vi "FPGA_main_simplified.vi"() -> ()   [LabVIEW 2020]
uses:
  <vilib>/Platform/TimedLoop/XDataNode/timing_clust.ctl
  <vilib>/Platform/TimedLoop/XDataNode/nitl_modes.ctl
  <vilib>/Platform/TimedLoop/XDataNode/wakeup.ctl
  <vilib>/LabVIEW Targets/FPGA/cRIO/shared/nicrio_ModuleControls/nicrio_cRIO-9775_ContinuousDataRates4ChansRing.ctl
  <vilib>/rvi/Emulation/niFpgaGetClockAttributes.vi
  <vilib>/rvi/Emulation/niFpgaSctlEmulationGetInTimedLoop.vi
  <vilib>/rvi/Emulation/niFpgaEmulationReportErrorSimple.vi
  <vilib>/rvi/Emulation/niFpgaProcessEmulError.vi
  <vilib>/rvi/Emulation/niFpgaCriticalErrorInLSC.vi
  <vilib>/rvi/eio/common/nirviEmuTemplateMethod_errors.vi
  <vilib>/rvi/eio/common/nirviEmuTemplatePropertySet_errors.vi
  <vilib>/rvi/interface/RandomDataEmulation/niFpgaRandomDataHandleErrors.vi
  <vilib>/platform/TimedLoop/XDataNode/XDataNode.xnode
  <vilib>/eio/EIONode/EIONode.xnode
  <vilib>/eio/EIOMethodNode/EIOMethodNode.xnode
  <vilib>/eio/EIOPropertyNode/EIOPropertyNode.xnode
  <vilib>/rvi/DataTransferAndStorage/Container/XNode/niFpgaContainer.xnode
  <vilib>/rvi/interface/RandomDataEmulation/nirviRandomDataFpgaReadWriteTemplate.vi
  <vilib>/Platform/TimedLoop/XDataNode/XDNodeRunTimeDep.lvlib
  <vilib>/rvi/eio/common/nirviEmuTemplatePropertyGet_errors.vi
  <vilib>/rvi/eio/common/nirviEmuTemplatePropertyGet_noerrors.vi
  <vilib>/rvi/eio/common/nirviEmuTemplatePropertySet_noerrors.vi
panel:
  out "FPGA routine\nrunning":bool
  in  "Pulse\nWidth":u32 caption="Pulse width(uSec)"
  in  "Pulse\nPeriod":u32 caption="Period(uSec)"
  in  "Stop Routine":bool
  in  "DIO3":bool
  in  "DIO2":bool
  in  "DIO1":bool
  in  "DIO0":bool
  out "Rebinned Counts":i32
  in  "Binning Time (ticks)":i32=1200000
  out "Counts":u8
  out "FPGA Error":errorcluster
  out "Finished":bool
  in  "Stop":bool
  out "Module Underflow":bool
  out "DMA FIFO Full":bool
  out "Actual Loop Period (ticks)":u32=40
  out "First Read":bool
  in  "Type Counter":enum16{"Falling Edge", "Rising Edge"}(ring)
  # "Photon counting. Single cycle time loop"
  # "User Control of digital output"
  # "Thresholding"
  # "Pulsing DIO 0 (Pulse width should be shorter than\n period)"
  # "Binning and streaming binned Total Count"
  # "Streaming Analog Input Data"
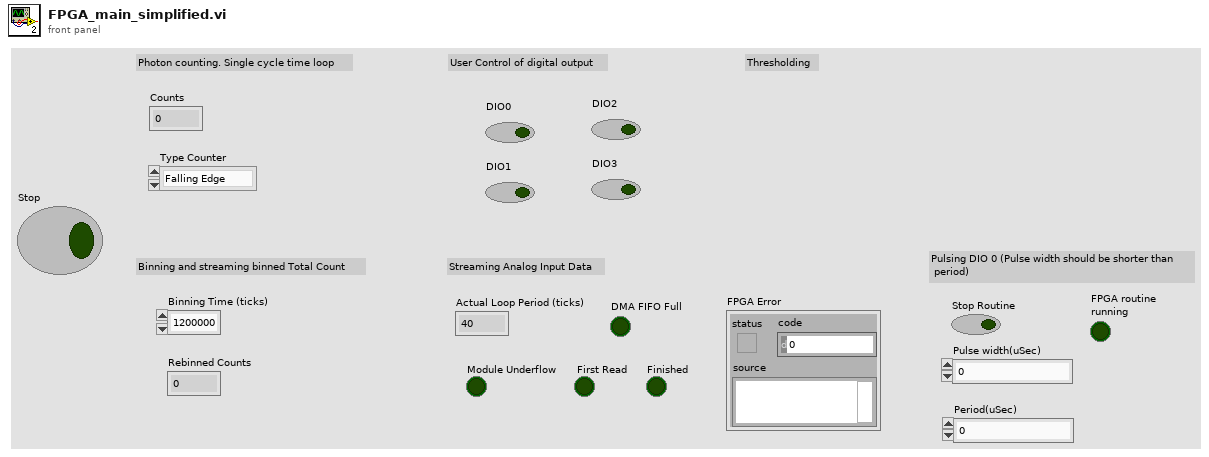
[diagram p1: front panel]
types:
  T1 = typedef "nicrio_cRIO-9775_ContinuousDataRates4ChansRing.ctl" = u16
  T2 = typedef "XDNodeRunTimeDep.lvlib/timing_clust.ctl" = cluster{"Expected End [f-1]":u64, "Actual End [f-1]":u64, "Finished Late? [f-1]":bool, "Expected End [i-1]":u64, "Actual End [i-1]":u64, "Finished Late? [i-1]":bool, "Expected Start [i]":u64, "Actual Start [i]":u64, "Expected Start [f]":u64, "Actual Start [f]":u64, "Source Name":string, "Structure Name":string, "Period":i64, "Deadline":i64, "Offset":i64, "Start":i64, "Priority":i32, "Timeout":i32, "Mode":T3, "Wakeup Reason":T4, "Error":errorcluster, "Source Type":string, "Secondary Source Type":string, "Global End Time":u64, "Global Start Time":u64, "Frame Duration":u64, "Iteration Duration":u64, "Assigned CPU":i32, "I/O Scan Engine Mode":u32}
  T3 = typedef "XDNodeRunTimeDep.lvlib/nitl_modes.ctl" = enum32{"No Change", "Process missed periods, maintain original phase", "Discard missed periods, maintain original phase", "Process missed periods, ignore original phase", "Discard missed periods, ignore original phase"}
  T4 = typedef "XDNodeRunTimeDep.lvlib/wakeup.ctl" = enum32{"Normal", "Aborted", "Asynchronous wakeup", "Timing source error", "Timed loop error", "Timeout"}
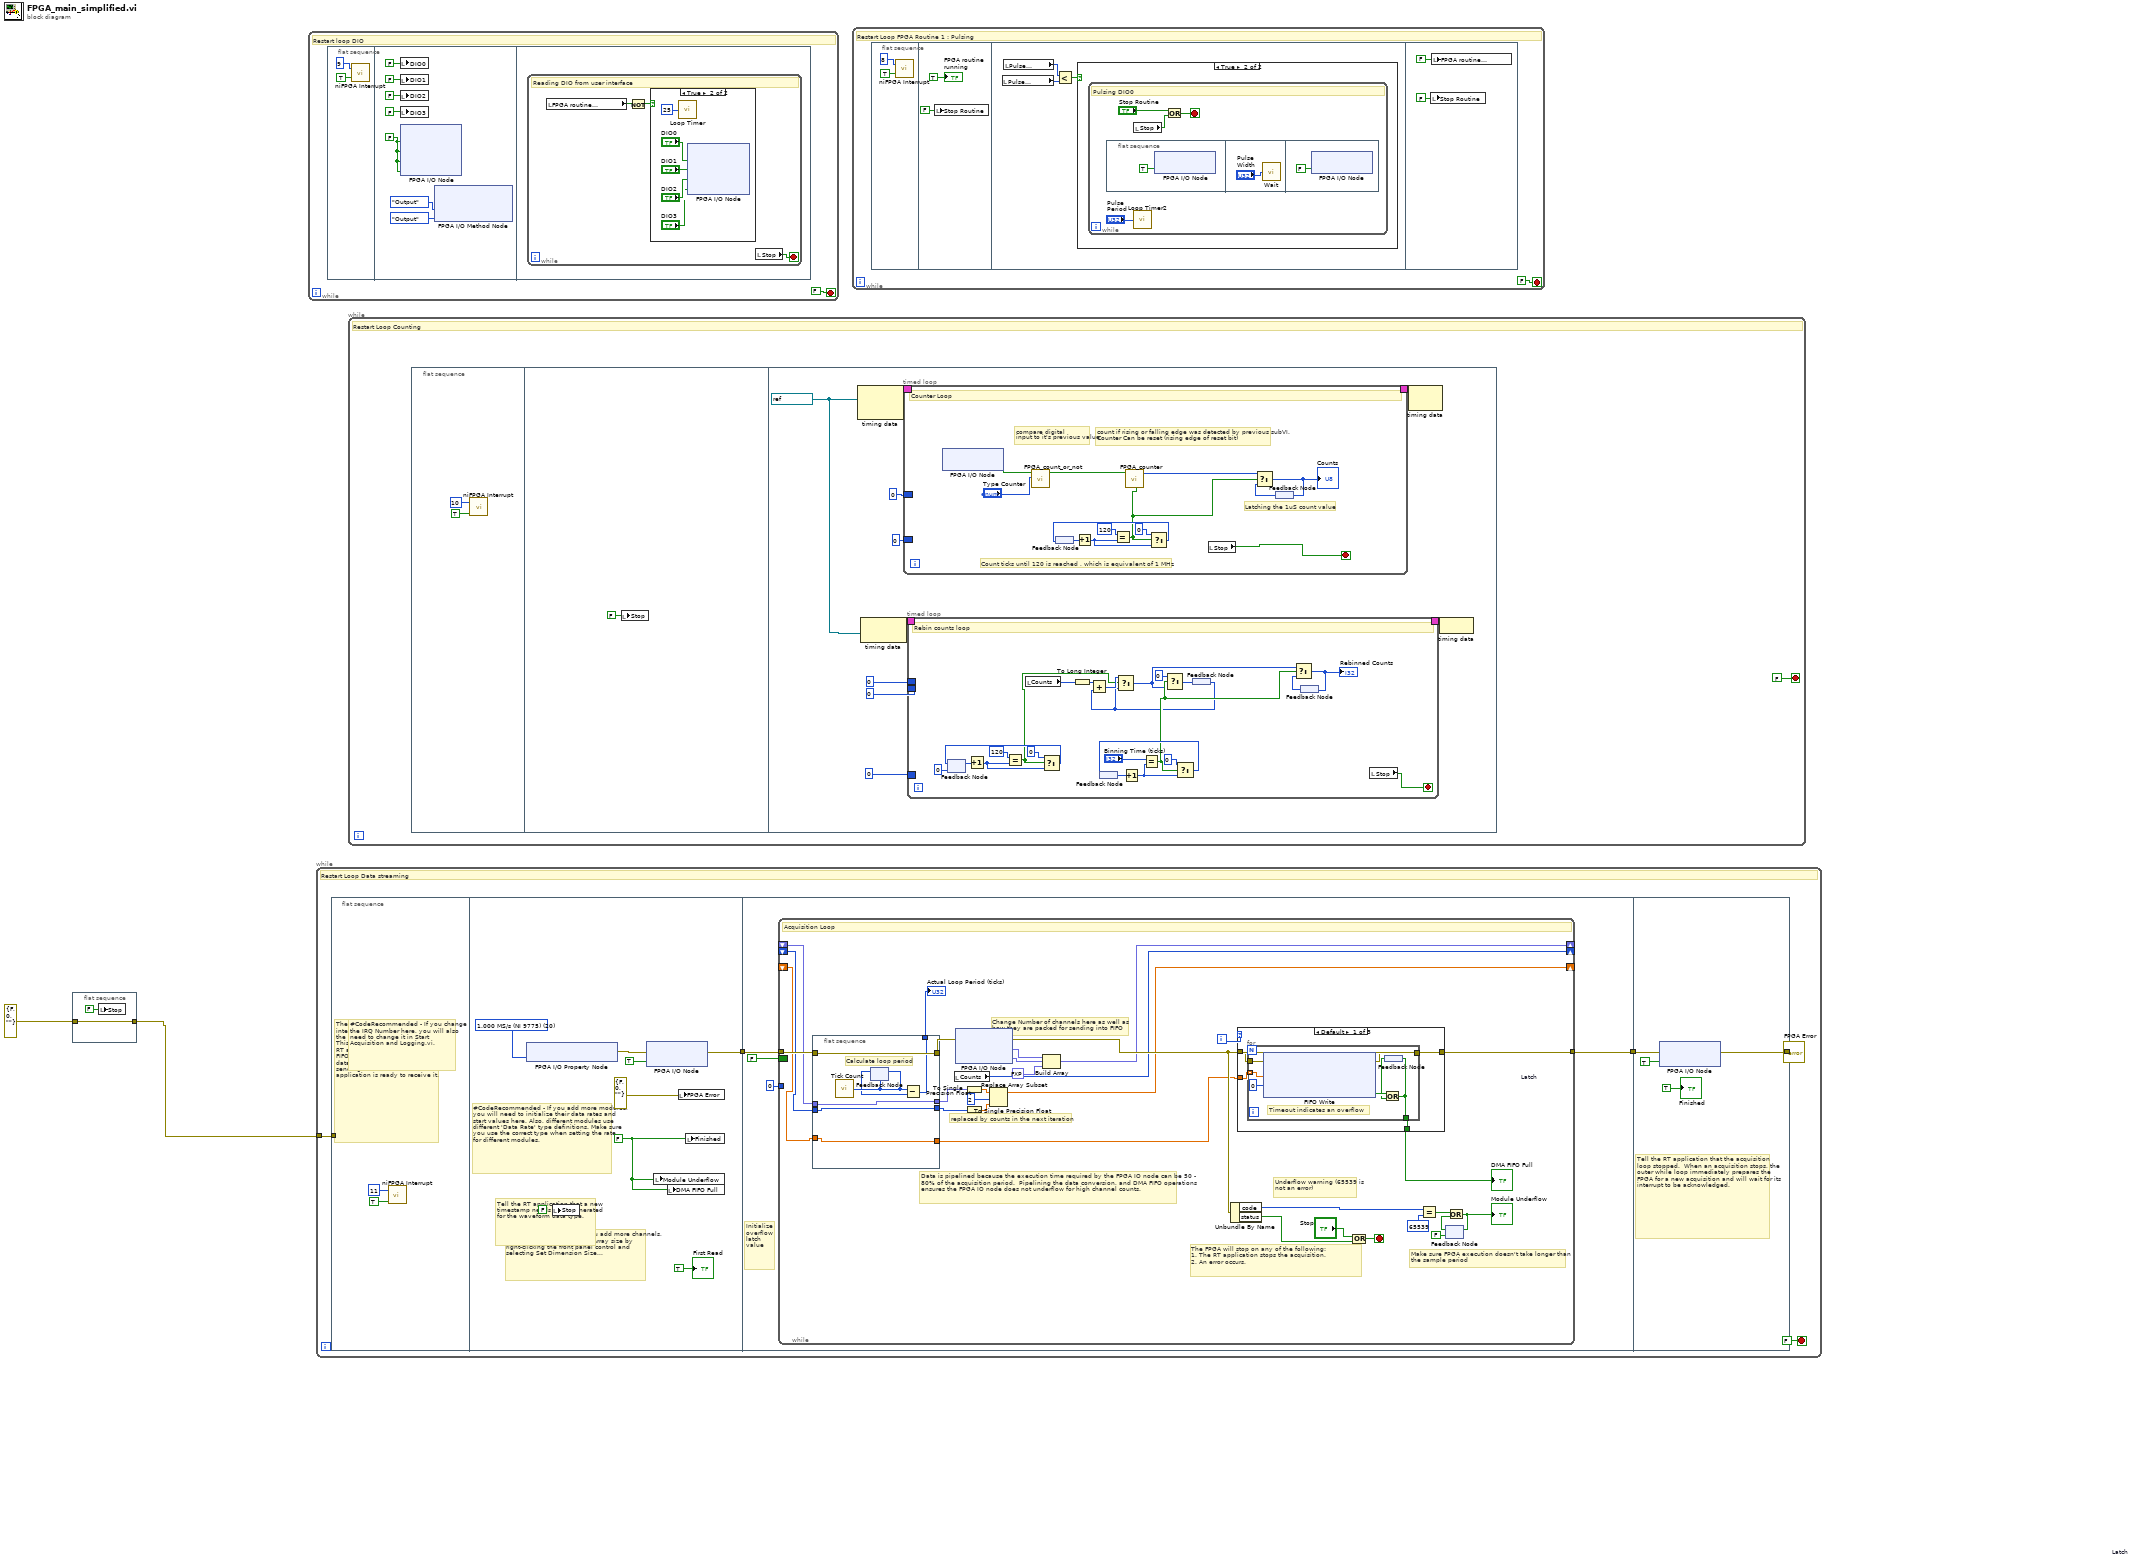
[diagram p0: block diagram]
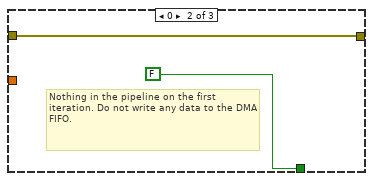
[diagram p4: hidden frame]
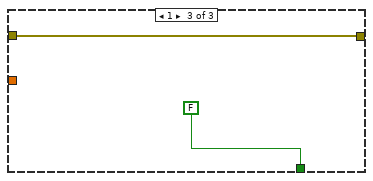
[diagram p5: hidden frame]
diagram:
  n1 = flat-sequence {
    tunnel: errorcluster {"status"=FALSE, "code"=0, "source"=""} ("Error") -> [w3]
    tunnel: [w3] -> w1
    frame #0 {
      n2 = local write "Stop"(FALSE ("stop")) -> ()
    }
  }
  n3 = while {
    stop <- FALSE stop-if-true
    # "Restart loop DIO"
    n4 = flat-sequence {
      frame #0 {
        n5 = call <vilib>:"niFPGA Interrupt.vi"("Wait Until Cleared (F)"=TRUE ("Wait Until Cleared"), "IRQ Number (0)"=u8 9 ("IRQ Number")) -> ()  [unwired: 1 in]
      }
      frame #1 {
        w10 = FALSE ("Mod3/DIO0")
        n6 = local write "DIO0"(FALSE ("DIO0")) -> ()
        n7 = local write "DIO1"(FALSE ("DIO1")) -> ()
        n8 = local write "DIO2"(FALSE ("DIO2")) -> ()
        n9 = local write "DIO3"(FALSE ("DIO3")) -> ()
        n10 = xnode "FPGA I/O Node"("Mod3/DIO0"=w10, "Mod3/DIO1"=w10, "Mod3/DIO2"=w10, "Mod3/DIO3"=w10) -> ()  [unwired: 4 in, 4 out]
        n11 = xnode "FPGA I/O Method Node"("DIO 7:4"=enum8{"No Change", "Input", "Output"}."Output", "DIO 3:0"=enum8{"No Change", "Input", "Output"}."Output") -> ()  [unwired: 1 in, 1 out]
      }
      frame #2 {
        n12 = while {
          stop <- w17 stop-if-true
          # "Reading DIO from user interface"
          n13 = local read "FPGA routine\nrunning"() -> (w16:bool)
          n14 = Not(x=w16) -> (.not. x?=w15:bool)
          n15 = case shown="True" w15 {
            frame False {
            }
            frame True {
              n16 = call "Loop Timer"("Count(mSec)"=u8 25) -> ()  [unwired: 1 out]
              n17 = xnode "FPGA I/O Node"("Mod3/DIO0"="DIO0", "Mod3/DIO1"="DIO1", "Mod3/DIO2"="DIO2", "Mod3/DIO3"="DIO3") -> ()  [unwired: 4 in, 4 out]
            }
          }
          n18 = local read "Stop"() -> (w17:bool)
        }
      }
    }
  }
  n19 = while {
    tunnel: w1 -> [w23]
    stop <- FALSE stop-if-true
    # "Restart Loop Data streaming"
    n20 = flat-sequence {
      tunnel: w23 -> [_]
      tunnel: [w37] -> w26
      tunnel: w26 -> [w39]
      tunnel: [w38] -> w25
      tunnel: w25 -> [w96]
      tunnel: [w95] -> w24
      frame #0 {
        # "#CodeRecommended - If you change the IRQ Number here, you will also need to change it in Start Acquisition and Logging.vi."
        # "The RT application waits on this interrupt to synchronize itself with the start of the FPGA's acquisition.  This synchronization prevents the RT application from polling the DMA FIFO before the FPGA is sending its data. It also prevents the FPGA from sending its data before the RT application is ready to receive it."
        n21 = call <vilib>:"niFPGA Interrupt.vi"("Wait Until Cleared (F)"=TRUE ("Wait Until Cleared"), "IRQ Number (0)"=u8 11 ("IRQ Number")) -> ()  [unwired: 1 in]
      }
      frame #1 {
        w31 = T1 20 items=["1.000 MS/s (NI 9775)"=20, "833.333 KS/s (NI 9775)"=24, "714.286 KS/s (NI 9775)"=28, "625.000 KS/s (NI 9775)"=32, "555.556 KS/s (NI 9775)"=36, "500.000 KS/s (NI 9775)"=40, "454.545 KS/s (NI 9775)"=44, "416.667 KS/s (NI 9775)"=48, "384.615 KS/s (NI 9775)"=52, "357.143 KS/s (NI 9775)"=56, "333.333 KS/s (NI 9775)"=60, "312.500 KS/s (NI 9775)"=64, "294.118 KS/s (NI 9775)"=68, "277.778 KS/s (NI 9775)"=72, "263.158 KS/s (NI 9775)"=76, "250.000 KS/s (NI 9775)"=80, "238.095 KS/s (NI 9775)"=84, "227.273 KS/s (NI 9775)"=88, "217.391 KS/s (NI 9775)"=92, "208.333 KS/s (NI 9775)"=96, "200.000 KS/s (NI 9775)"=100, "192.308 KS/s (NI 9775)"=104, "185.185 KS/s (NI 9775)"=108, "178.571 KS/s (NI 9775)"=112, "172.414 KS/s (NI 9775)"=116, "166.667 KS/s (NI 9775)"=120, "161.290 KS/s (NI 9775)"=124, "156.250 KS/s (NI 9775)"=128, "151.515 KS/s (NI 9775)"=132, "147.059 KS/s (NI 9775)"=136, "142.857 KS/s (NI 9775)"=140, "138.889 KS/s (NI 9775)"=144, "135.135 KS/s (NI 9775)"=148, "131.579 KS/s (NI 9775)"=152, "128.205 KS/s (NI 9775)"=156, "125.000 KS/s (NI 9775)"=160, "121.951 KS/s (NI 9775)"=164, "119.048 KS/s (NI 9775)"=168, "116.279 KS/s (NI 9775)"=172, "113.636 KS/s (NI 9775)"=176, "111.111 KS/s (NI 9775)"=180, "108.696 KS/s (NI 9775)"=184, "106.383 KS/s (NI 9775)"=188, "104.167 KS/s (NI 9775)"=192, "102.041 KS/s (NI 9775)"=196, "100.000 KS/s (NI 9775)"=200, "50.000 KS/s (NI 9775)"=400, "33.333 KS/s (NI 9775)"=600, "25.000 KS/s (NI 9775)"=800, "20.000 KS/s (NI 9775)"=1000, "16.667 KS/s (NI 9775)"=1200, "14.286 KS/s (NI 9775)"=1400, "12.500 KS/s (NI 9775)"=1600, "11.111 KS/s (NI 9775)"=1800, "10.000 KS/s (NI 9775)"=2000, "9.091 KS/s (NI 9775)"=2200, "8.333 KS/s (NI 9775)"=2400, "7.692 KS/s (NI 9775)"=2600, "7.143 KS/s (NI 9775)"=2800, "6.667 KS/s (NI 9775)"=3000, "6.250 KS/s (NI 9775)"=3200, "5.882 KS/s (NI 9775)"=3400, "5.556 KS/s (NI 9775)"=3600, "5.000 KS/s (NI 9775)"=4000, "4.762 KS/s (NI 9775)"=4200, "4.545 KS/s (NI 9775)"=4400, "4.348 KS/s (NI 9775)"=4600, "4.167 KS/s (NI 9775)"=4800, "4.000 KS/s (NI 9775)"=5000, "3.846 KS/s (NI 9775)"=5200, "3.571 KS/s (NI 9775)"=5600, "3.333 KS/s (NI 9775)"=6000, "3.125 KS/s (NI 9775)"=6400, "2.941 KS/s (NI 9775)"=6800, "2.778 KS/s (NI 9775)"=7200, "2.632 KS/s (NI 9775)"=7600, "2.500 KS/s (NI 9775)"=8000, "2.381 KS/s (NI 9775)"=8400, "2.273 KS/s (NI 9775)"=8800, "2.174 KS/s (NI 9775)"=9200, "2.083 KS/s (NI 9775)"=9600, "2.000 KS/s (NI 9775)"=10000, "1.923 KS/s (NI 9775)"=10400, "1.852 KS/s (NI 9775)"=10800, "1.786 KS/s (NI 9775)"=11200, "1.724 KS/s (NI 9775)"=11600, "1.667 KS/s (NI 9775)"=12000, "1.613 KS/s (NI 9775)"=12400, "1.563 KS/s (NI 9775)"=12800, "1.515 KS/s (NI 9775)"=13200, "1.471 KS/s (NI 9775)"=13600, "1.429 KS/s (NI 9775)"=14000, "1.389 KS/s (NI 9775)"=14400, "1.351 KS/s (NI 9775)"=14800, "1.316 KS/s (NI 9775)"=15200, "1.282 KS/s (NI 9775)"=15600, "1.250 KS/s (NI 9775)"=16000, "1.220 KS/s (NI 9775)"=16400, "1.190 KS/s (NI 9775)"=16800, "1.163 KS/s (NI 9775)"=17200, "1.136 KS/s (NI 9775)"=17600, "1.111 KS/s (NI 9775)"=18000, "1.087 KS/s (NI 9775)"=18400, "1.064 KS/s (NI 9775)"=18800, "1.042 KS/s (NI 9775)"=19200, "1.020 KS/s (NI 9775)"=19600, "1.000 KS/s (NI 9775)"=20000, "0.980 KS/s (NI 9775)"=20400, "0.962 KS/s (NI 9775)"=20800, "0.943 KS/s (NI 9775)"=21200, "0.926 KS/s (NI 9775)"=21600, "0.909 KS/s (NI 9775)"=22000, "0.893 KS/s (NI 9775)"=22400, "0.877 KS/s (NI 9775)"=22800, "0.862 KS/s (NI 9775)"=23200, "0.847 KS/s (NI 9775)"=23600, "0.833 KS/s (NI 9775)"=24000, "0.820 KS/s (NI 9775)"=24400, "0.806 KS/s (NI 9775)"=24800, "0.794 KS/s (NI 9775)"=25200, "0.781 KS/s (NI 9775)"=25600, "0.694 KS/s (NI 9775)"=28800, "0.625 KS/s (NI 9775)"=32000, "0.568 KS/s (NI 9775)"=35200, "0.521 KS/s (NI 9775)"=38400, "0.446 KS/s (NI 9775)"=44800, "0.391 KS/s (NI 9775)"=51200, "0.347 KS/s (NI 9775)"=57600, "0.313 KS/s (NI 9775)"=64000] ("Continuous Data Rate")
        w34 = FALSE ("Module Underflow")
        # "Tell the RT application that a new timestamp needs to be generated for the waveform data type."
        # "#CodeRecommended - If you add more channels, increase the Channel Scale Array size by right-clicking the front panel control and selecting Set Dimension Size..."
        # "#CodeRecommended - If you add more modules, you will need to initialize their data rates and start values here. Also, different modules use different 'Data Rate' type definitions. Make sure you use the correct type when setting the rate for different modules."
        n22 = xnode "FPGA I/O Property Node"("Continuous Data Rate"=w31) -> ("error out"=w33:errorcluster)  [unwired: 2 in, 1 out]
        n23 = local write "Stop"(FALSE ("Stop")) -> ()
        n24 = xnode "FPGA I/O Node"("error in"=w33, "Mod1/Start"=TRUE) -> ("error out"=w37:errorcluster)  [unwired: 1 in, 1 out]
        n25 = local write "Module Underflow"(w34) -> ()
        n26 = local write "DMA FIFO Full"(w34) -> ()
        n27 = local write "FPGA Error"(errorcluster {"status"=FALSE, "code"=0, "source"=""} ("FPGA Error")) -> ()
        n28 = local write "Finished"(w34) -> ()
        "First Read" <- TRUE ("First Read")
      }
      frame #2 {
        # "Initialize overflow latch value"
        n29 = while {
          tunnel: w39 -> [w67]
          tunnel: [w72] -> w38
          border: FALSE ("Overflow\nLatch") -> [_]
          tunnel: u8 0 ("Counts") -> [_]
          shift-right: [w55] -> _
          shift-left: _ -> [w54]
          shift-right: [w44] -> _
          shift-left: _ -> [w52]
          shift-right: [w50] -> _
          shift-left: _ -> [w49]
          i -> [w58]
          stop <- w71 stop-if-true
          # "replaced by counts in the next iteration"
          # "Data is pipelined because the execution time required by the FPGA IO node can be 50 - 80% of the acquisition period.  Pipelining the data conversion, and DMA FIFO operations ensures the FPGA IO node does not underflow for high channel counts."
          # "Change Number of channels here as well as \nhow they are packed for sending into FIFO"
          # "Underflow warning (65539 is not an error)"
          # "The FPGA will stop on any of the following:\n1. The RT application stops the acquisition.\n2. An error occurs."
          # "Make sure FPGA execution doesn't take longer than the sample period"
          # "Acquisition Loop"
          n30 = flat-sequence {
            tunnel: [w94] -> w66
            tunnel: w67 -> [w94]
            tunnel: [w91] -> w65
            tunnel: w54 -> [w90]
            tunnel: [w90] -> w53
            tunnel: w52 -> [w89]
            tunnel: [w89] -> w51
            tunnel: w49 -> [w88]
            tunnel: [w88] -> w48
            frame #0 {
              # "Calculate loop period"
              n31 = call "Tick Count"() -> ("Tick Count(Ticks)"=w93:u32)
              n32 = feedback-in #1(w93) -> ()
              n33 = feedback #1(w93) -> (w92:u32)
              n34 = Subtract(x=w93, y=w92) -> (x-y=w91:u32)
            }
          }
          n35 = local read "Counts"() -> (w50:u8)
          n36 = xnode "FPGA I/O Node"("error in"=w66) -> ("error out"=w56:errorcluster, "Mod1/AI0"=w43:fxp<+/-,17,5>, "Mod1/AI1"=w42:fxp<+/-,17,5>)  [unwired: 2 in, 2 out]
          n37 = To Single Precision Float(number=w53) -> (single precision float=w47:sgl[])
          n38 = To Single Precision Float(number=w48) -> (single precision float=w45:sgl)
          n39 = Replace Array Subset(array=w47, new element=w45, index=2) -> (w44:sgl[])
          n40 = Build Array(w43, w42, fxp<+/-,17,5> 0.0 ("element")) -> (w55:fxp<+/-,17,5>[])
          n41 = case shown="Default" w58 {
            tunnel: [w73 FALSE FALSE] -> w68
            tunnel: w51 -> [w76 _ _]
            tunnel: w56 -> [w75 w84 w86]
            tunnel: [w74 w84 w86] -> w72
            frame Default {
              n42 = for {
                tunnel: [w81] -> w73
                tunnel: w76 -> [w77] mode=indexing
                tunnel: w75 -> [w79]
                tunnel: [w78] -> w74
                # "Timeout indicates an overflow"
                n43 = xnode ("FIFO Write")("Element"=w77, "Timeout"=0, "error in (no error)"=w79) -> ("Timed Out?"=w83:bool, "error out"=w78:errorcluster)  [unwired: 1 in, 1 out]
                n44 = feedback #2 "Latch"() -> (w82:bool)
                n45 = Or(x=w83, y=w82) -> (x .or. y?=w81:bool)
                n46 = feedback-in #2(w81) -> ()
              }
            }
            frame 0 {
              # "Nothing in the pipeline on the first iteration. Do not write any data to the DMA FIFO."
            }
            frame 1 {
            }
          }
          "DMA FIFO Full" <- w68
          n47 = Unbundle By Name(w72) -> ("code"=w69:i32, "status"=w60:bool)
          n48 = Compound Arithmetic op=OR("Stop", w60) -> (w71:bool)
          n49 = Equal?(x=w69, y=65539) -> (x = y?=w62:bool)
          n50 = feedback #3 "Latch"(FALSE) -> (w64:bool)
          n51 = Or(x=w62, y=w64) -> (x .or. y?=w61:bool)
          "Module Underflow" <- w61
          n52 = feedback-in #3(w61) -> ()
          "Actual Loop Period (ticks)" <- w65
        }
      }
      frame #3 {
        # "Tell the RT application that the acquisition loop stopped.  When an acquisition stops, the outer while loop immediately prepares the FPGA for a new acquisition and will wait for its interrupt to be acknowledged."
        n53 = xnode "FPGA I/O Node"("error in"=w96, "Mod1/Stop"=TRUE) -> ("error out"=w95:errorcluster)  [unwired: 1 in, 1 out]
        "Finished" <- TRUE ("Finished")
      }
    }
    "FPGA Error" <- w24
  }
  n54 = while {
    stop <- FALSE stop-if-true
    # "Restart Loop Counting"
    n55 = flat-sequence {
      frame #0 {
        n56 = call <vilib>:"niFPGA Interrupt.vi"("Wait Until Cleared (F)"=TRUE ("Wait Until Cleared"), "IRQ Number (0)"=u8 10 ("IRQ Number")) -> ()  [unwired: 1 in]
      }
      frame #1 {
        n57 = local write "Stop"(FALSE ("Stop")) -> ()
      }
      frame #2 {
        w105 = refnum<k21> "120MHz" ("Source Name")
        n58 = node-c288(w105) -> (w112:T2)  [unwired: 1 in]
        n59 = node-c288(w105) -> (w108:T2)
        n60 = timed-loop {
          timing: w112 -> [_]
          timing-out: [_] -> w111
          border: u8 0 ("t") -> [_]
          border: u8 0 ("Total Count") -> [_]
          stop <- w142 stop-if-true
          # "Latching the 1uS count value"
          # "Count ticks until 120 is reached , which is equivalent of 1 MHz"
          # "count if rising or falling edge was detected by previous subVI. Counter Can be reset (rising edge of reset bit)"
          # "compare digital\ninput to it's previous value"
          # "Counter Loop"
          n61 = xnode "FPGA I/O Node"() -> ("Mod2/DIO0"=w153:bool)  [unwired: 1 in, 1 out]
          n62 = call "FPGA_count_or_not.vi"("Type Counter"="Type Counter", "Countable"=w153) -> ("Count or Not?"=w154:bool)  [unwired: 9 in]
          n63 = feedback #4() -> (w151:u8)
          n64 = Increment(x=w151) -> (x+1=w149:u8)
          n65 = Equal?(x=u8 120 ("y"), y=w149) -> (x = y?=w146:bool)
          n66 = call "FPGA_counter.vi"("Count or Not?"=w154, "Reset Photon Count"=w146) -> ("Total Count"=w145:u8)  [unwired: 8 in]
          n67 = Select(t=u8 0, s=w146, f=w149) -> (s? t:f=w147:u8)
          n68 = feedback-in #4(w147) -> ()
          n69 = local read "Stop"() -> (w142:bool)
          n70 = feedback #5() -> (w143:u8)
          n71 = Select(t=w145, s=w146, f=w143) -> (s? t:f=w144:u8)
          "Counts" <- w144
          n72 = feedback-in #5(w144) -> ()
        }
        n73 = timed-loop {
          timing: w108 -> [_]
          timing-out: [_] -> w107
          border: 0 ("Counts") -> [_]
          border: 0 ("t") -> [_]
          border: 0 -> [_]
          stop <- w125 stop-if-true
          # "Rebin counts loop"
          n74 = feedback #6(u8 0 ("t")) -> (w122:u8)
          n75 = Increment(x=w122) -> (x+1=w120:u8)
          n76 = Equal?(x=u8 120 ("y"), y=w120) -> (x = y?=w115:bool)
          n77 = local read "Counts"() -> (w124:u8)
          n78 = Select(t=u8 0, s=w115, f=w120) -> (s? t:f=w118:u8)
          n79 = feedback-in #6(w118) -> ()
          n80 = To Long Integer(number=w124) -> (32bit integer=w123:i32)
          n81 = feedback #7() -> (w132:i32)
          n82 = Increment(x=w132) -> (x+1=w133:i32)
          n83 = Equal?(x="Binning Time (ticks)", y=w133) -> (x = y?=w128:bool)
          n84 = Select(t=0, s=w128, f=w133) -> (s? t:f=w135:i32)
          n85 = feedback-in #7(w135) -> ()
          n86 = feedback #8() -> (w116:i32)
          n87 = Add(x=w123, y=w116) -> (x+y=w117:i32)
          n88 = Select(t=w117, s=w115, f=w116) -> (s? t:f=w113:i32)
          n89 = Select(t=0, s=w128, f=w113) -> (s? t:f=w127:i32)
          n90 = feedback-in #8(w127) -> ()
          n91 = feedback #9() -> (w129:i32)
          n92 = Select(t=w113, s=w128, f=w129) -> (s? t:f=w130:i32)
          "Rebinned Counts" <- w130
          n93 = feedback-in #9(w130) -> ()
          n94 = local read "Stop"() -> (w125:bool)
        }
        n95 = node-c288(w111) -> ()  [unwired: 1 out]
        n96 = node-c288(w107) -> ()
      }
    }
  }
  n97 = while {
    stop <- FALSE stop-if-true
    # "Restart Loop FPGA Routine 1 : Pulsing"
    n98 = flat-sequence {
      frame #0 {
        n99 = call <vilib>:"niFPGA Interrupt.vi"("Wait Until Cleared (F)"=TRUE ("Wait Until Cleared"), "IRQ Number (0)"=u8 8 ("IRQ Number")) -> ()  [unwired: 1 in]
      }
      frame #1 {
        n100 = local write "Stop Routine"(FALSE ("Stop Routine")) -> ()
        "FPGA routine\nrunning" <- TRUE
      }
      frame #2 {
        n101 = local read "Pulse\nPeriod"() -> (w167:u32)
        n102 = local read "Pulse\nWidth"() -> (w168:u32)
        n103 = Less?(x=w168, y=w167) -> (x < y?=w166:bool)
        n104 = case shown="True" w166 {
          frame False {
          }
          frame True {
            n105 = while {
              stop <- w171 stop-if-true
              # "Pulsing DIO0"
              n106 = flat-sequence {
                frame #0 {
                  n107 = xnode "FPGA I/O Node"("Mod3/DIO0"=TRUE) -> ()  [unwired: 1 in, 1 out]
                }
                frame #1 {
                  n108 = call "Wait"("Count(uSec)"="Pulse\nWidth") -> ()  [unwired: 1 out]
                }
                frame #2 {
                  n109 = xnode "FPGA I/O Node"("Mod3/DIO0"=FALSE) -> ()  [unwired: 1 in, 1 out]
                }
              }
              n110 = local read "Stop"() -> (w172:bool)
              n111 = call "Loop Timer2"("Count(uSec)"="Pulse\nPeriod") -> ()  [unwired: 1 out]
              n112 = Or(x="Stop Routine", y=w172) -> (x .or. y?=w171:bool)
            }
          }
        }
      }
      frame #3 {
        n113 = local write "Stop Routine"(FALSE ("Stop Routine")) -> ()
        n114 = local write "FPGA routine\nrunning"(FALSE ("FPGA routine\nrunning")) -> ()
      }
    }
  }
